vi "Start.vi"(8 "error in (no error)":errorcluster, 11 "Module Config Selector":i16) -> (0 "error out":errorcluster)   [LabVIEW 2017, in "BOP_VibAPI_2.lvlib"]
uses:
  <vilib>/addons/InsightCM/Devices/Shared/Cms/Fpga/Acquisition/source/subVIs/VibAPI_2/BOP_VibAPI_2.lvlib
  <vilib>/rvi/eio/common/nirviEmuTemplateMethod_errors.vi
  <vilib>/eio/EIONode/EIONode.xnode
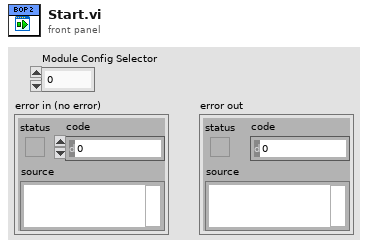
[diagram p1: front panel]
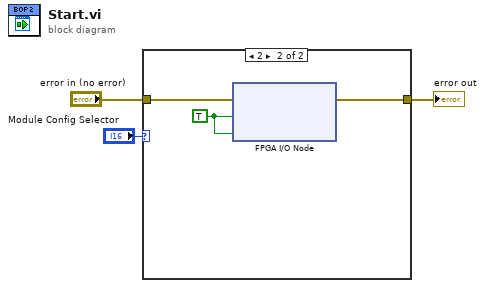
[diagram p0: block diagram]
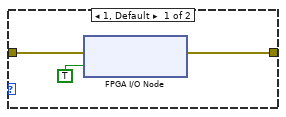
[diagram p2: hidden frame]
diagram:
  n1 = case shown="2" "Module Config Selector" {
    tunnel: "error in (no error)" -> [w5 w8]
    tunnel: [w6 w9] -> w2
    frame 1, Default {
      n2 = xnode "FPGA I/O Node"("error in"=w5, "Mod1/Start"=TRUE) -> ("error out"=w6:errorcluster)  [unwired: 1 in, 1 out]
    }
    frame 2 {
      w7 = TRUE
      n3 = xnode "FPGA I/O Node"("error in"=w8, "Mod1/Start"=w7, "Mod2/Start"=w7) -> ("error out"=w9:errorcluster)  [unwired: 2 in, 2 out]
    }
  }
  "error out" <- w2
